vi "Untitled 1.vi"(8 "error in (no error)":errorcluster, 11 "Abstract Log Producer in":refnum<class "Abstract Log Producer.lvclass">) -> (0 "error out":errorcluster, 3 "Abstract Log Producer out":refnum<class "Abstract Log Producer.lvclass">)   [LabVIEW 2020, in "Messaging.lvlib" / "Abstract Log Producer.lvclass"]
uses:
  Abstract Log Producer.lvclass
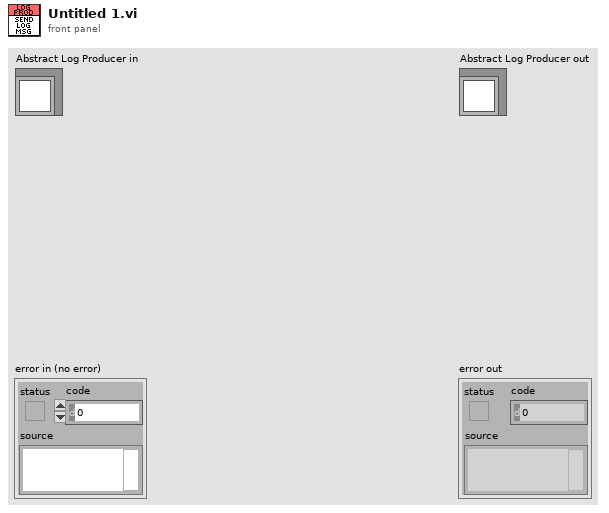
[diagram p1: front panel]
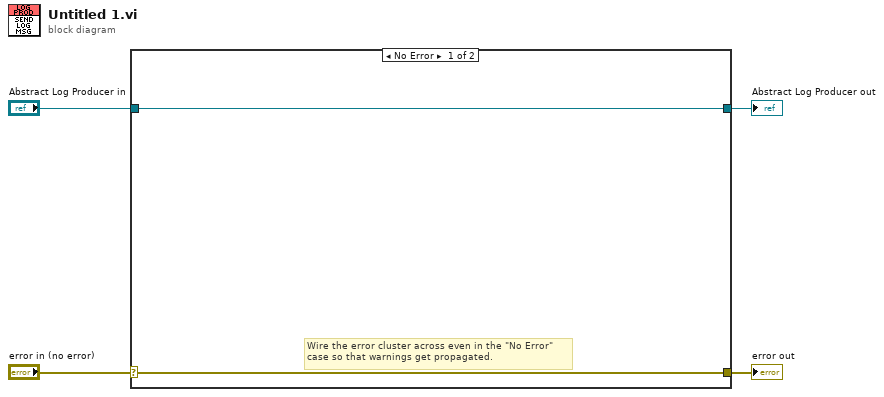
[diagram p0: block diagram]
diagram:
  n1 = case shown="No Error" "error in (no error)" {
    selector: "error in (no error)" -> [w5 w8]
    tunnel: [w5 w8] -> w3
    tunnel: [w6 w7] -> w1
    tunnel: "Abstract Log Producer in" -> [w6 w7]
    frame No Error {
      # "Wire the error cluster across even in the \"No Error\"\ncase so that warnings get propagated."
    }
    frame Error {
    }
  }
  "error out" <- w3
  "Abstract Log Producer out" <- w1
